vi "Periodic Tasks Gear.vi"(8 "error in":errorcluster) -> ()   [LabVIEW 2016]
uses:
  <userlib>/836-libraries/Drive/Drive_Code/Drive_Code_Support/Drive_Code_PID_Bundle.ctl
  <vilib>/Platform/TimedLoop/XDataNode/timing_clust.ctl
  <vilib>/Platform/TimedLoop/XDataNode/nitl_modes.ctl
  <vilib>/Platform/TimedLoop/XDataNode/wakeup.ctl
  <vilib>/Rock Robotics/WPI/RobotDrive/WPI_RobotDriveDevRef.ctl
  <vilib>/Rock Robotics/WPI/MotorControl/WPI_MotorControlDeviceRef.ctl
  <vilib>/Rock Robotics/WPI/MotorControl/WPI_MotorControlType.ctl
  <vilib>/Rock Robotics/SystemInterfaces/DIO/FPGA_DIOPWMChannel.ctl
  <vilib>/Rock Robotics/WPI/PWM/WPI_PWMDeadband.ctl
  <vilib>/Rock Robotics/WPI/ThirdParty/CanMotor/TalonSRX/WPI_CANTalonSRX_APIControlMode.ctl
  <vilib>/Rock Robotics/WPI/Utilities/WPI_GetSetVariantRefNum.vi
  <vilib>/addons/control/pid/pid.llb/PID (DBL).vi
  <vilib>/platform/TimedLoop/XDataNode/XDataNode.xnode
  <vilib>/Platform/TimedLoop/XDataNode/XDNodeRunTimeDep.lvlib
  <vilib>/addons/control/pid/NI_PID_pid.lvlib
panel:
  in  "PID gains 2":T1={"proportional gain (Kc)"=0.08, "integral time (Ti, min)"=0.0, "derivative time (Td, min)"=0.001} {"derivative time (Td, min)" format="%.3f"; "integral time (Ti, min)" format="%.3f"; "proportional gain (Kc)" format="%.3f"}
  in  "Offset":dbl=30.0
  in  "Max Throttle":dbl=0.4
  in  "Negate":bool=TRUE
  in  "Follow Cam":bool=TRUE
  in  "reset":bool
  in  "PID Gains 2":T2={"Yaw, Driving Straight"={"proportional gain (Kc)"=0.035, "integral time (Ti, min)"=0.0, "derivative time (Td, min)"=0.0008}, "Yaw, Holding Still"={"proportional gain (Kc)"=0.0, "integral time (Ti, min)"=0.0, "derivative time (Td, min)"=0.0}, "Distance, Driving Straight"={"proportional gain (Kc)"=0.0, "integral time (Ti, min)"=0.0, "derivative time (Td, min)"=0.0}, "Distance, Holding Still"={"proportional gain (Kc)"=0.0, "integral time (Ti, min)"=0.0, "derivative time (Td, min)"=0.0}}
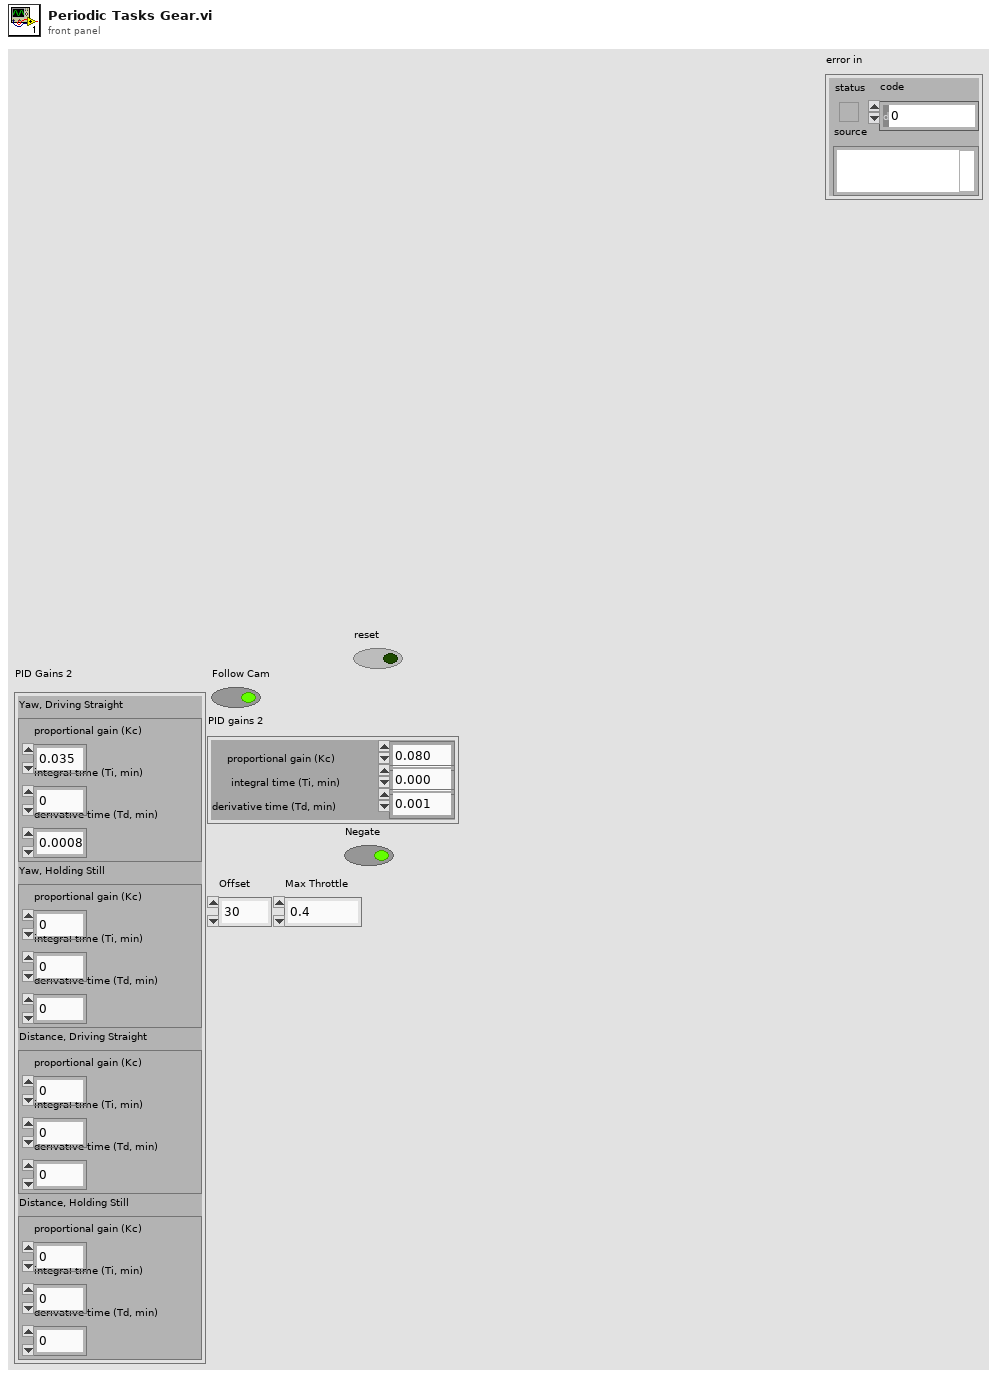
[diagram p1: front panel]
types:
  T1 = cluster{"proportional gain (Kc)":dbl, "integral time (Ti, min)":dbl, "derivative time (Td, min)":dbl}
  T2 = typedef "Drive_Code_PID_Bundle.ctl" = cluster{"Yaw, Driving Straight":cluster{"proportional gain (Kc)":dbl, "integral time (Ti, min)":dbl, "derivative time (Td, min)":dbl}, "Yaw, Holding Still":cluster{"proportional gain (Kc)":dbl, "integral time (Ti, min)":dbl, "derivative time (Td, min)":dbl}, "Distance, Driving Straight":cluster{"proportional gain (Kc)":dbl, "integral time (Ti, min)":dbl, "derivative time (Td, min)":dbl}, "Distance, Holding Still":cluster{"proportional gain (Kc)":dbl, "integral time (Ti, min)":dbl, "derivative time (Td, min)":dbl}}
  T3 = typedef "WPI_RobotDriveDevRef.ctl" = cluster{"DevStatus":errorcluster, "Motors[]":T4[], "Square Inputs":bool, "Max Output":dbl}
  T4 = typedef "WPI_MotorControlDeviceRef.ctl" = cluster{"DeviceStatus":errorcluster, "Type":T5, "PWM":cluster{"PWM Channel":T6, "DeadBand":T7}, "CAN":cluster{"Device Number":u8, "SetOutput VI Ref":variant, "GetOutput VI Ref":variant, "Enable VI Ref":variant, "Disable VI Ref":variant, "Data":variant}, "Invert":bool}
  T5 = typedef "WPI_MotorControlType.ctl" = enum16{"PWM", "CAN"}
  T6 = typedef "FPGA_DIOPWMChannel.ctl" = enum8{"PWM 0", "PWM 1", "PWM 2", "PWM 3", "PWM 4", "PWM 5", "PWM 6", "PWM 7", "PWM 8", "PWM 9", "PWM MXP 0", "PWM MXP 1", "PWM MXP 2", "PWM MXP 3", "PWM MXP 4", "PWM MXP 5", "PWM MXP 6", "PWM MXP 7", "PWM MXP 8", "PWM MXP 9", "Invalid"}
  T7 = typedef "WPI_PWMDeadband.ctl" = cluster{"Name":string, "maxPositivePwm":i32, "minPositivePwm":i32, "centerPwm":i32, "maxNegativePwm":i32, "minNegativePwm":i32, "angularRange":u16}
  T8 = typedef "Drive_Code_Bundle.ctl" = cluster{"Sensor Data":T9, "Drive Command rt fifo":refnum<k33>, "Logging Data":refnum<k33>}
  T9 = typedef "Sensor_Cluster.ctl" = cluster{"Gyro Data":cluster{"Gyro RT FIFO":refnum<k33>, "Gyro Current":dbl, "Gyro Hold":dbl}, "Encoder Data":cluster{"Encoder RT FIFO":refnum<k33>, "Encoder Current":dbl, "Encoder Hold":dbl}, "Camera Data":cluster{"Camera RT FIFO":refnum<k33>, "Camera Current":T10}}
  T10 = typedef "Camera_Cluster.ctl" = cluster{" Angle":dbl, "Valid":bool}
  T11 = typedef "WPI_EncoderDevRef.ctl" = cluster{"DevStatus":errorcluster, "EncoderIndex":T12, "CounterIndex":T13, "DistancePerCount":dbl, "Decoding Type":T14}
  T12 = typedef "FPGA_EncoderIdx.ctl" = enum8{"Enc 0", "Enc 1", "Enc 2", "Enc 3", "Enc 4", "Enc 5", "Enc 6", "Enc 7", "Invalid"}
  T13 = typedef "FPGA_CounterCtrSystemIndex.ctl" = enum8{"Ctr 0", "Ctr 1", "Ctr 2", "Ctr 3", "Ctr 4", "Ctr 5", "Ctr 6", "Ctr 7", "Invalid"}
  T14 = typedef "WPI_EncoderType.ctl" = enum16{"1x", "2x", "4x"}
  T15 = typedef "WPI_I2CDevRef.ctl" = cluster{"DevStatus":errorcluster, "Device Address":u8, "Handle":i32, "I2C Bus":T16}
  T16 = typedef "i2c_bus.ctl" = enum16{"I2C On-Board", "I2C MXP", "Invalid"}
  T17 = typedef "XDNodeRunTimeDep.lvlib/timing_clust.ctl" = cluster{"Expected End [f-1]":u64, "Actual End [f-1]":u64, "Finished Late? [f-1]":bool, "Expected End [i-1]":u64, "Actual End [i-1]":u64, "Finished Late? [i-1]":bool, "Expected Start [i]":u64, "Actual Start [i]":u64, "Expected Start [f]":u64, "Actual Start [f]":u64, "Source Name":string, "Structure Name":string, "Period":i64, "Deadline":i64, "Offset":i64, "Start":i64, "Priority":i32, "Timeout":i32, "Mode":T18, "Wakeup Reason":T19, "Error":errorcluster, "Source Type":string, "Secondary Source Type":string, "Global End Time":u64, "Global Start Time":u64, "Frame Duration":u64, "Iteration Duration":u64, "Assigned CPU":i32, "I/O Scan Engine Mode":u32}
  T18 = typedef "XDNodeRunTimeDep.lvlib/nitl_modes.ctl" = enum32{"No Change", "Process missed periods, maintain original phase", "Discard missed periods, maintain original phase", "Process missed periods, ignore original phase", "Discard missed periods, ignore original phase"}
  T19 = typedef "XDNodeRunTimeDep.lvlib/wakeup.ctl" = enum32{"Normal", "Aborted", "Asynchronous wakeup", "Timing source error", "Timed loop error", "Timeout"}
  T20 = typedef "WPI_JoystickDevRef.ctl" = cluster{"Device":T21}
  T21 = typedef "WPI_JoystickDeviceEnum.ctl" = enum16{"USB 0", "USB 1", "USB 2", "USB 3", "USB 4", "USB 5"}
  T22 = cluster{"Yaw":dbl, "Roll":dbl, "Pitch":dbl, "Yaw Wind":dbl, "Roll Wind":dbl, "Pitch Wind":dbl}
  T23 = typedef "WPI_CANTalonSRX_APIControlMode.ctl" = enum8{"Percent VBus", "Speed", "Position", "Slave", "Unchanged / Invalid", "Voltage Compensation", "Current", "Motion Profile", "Motion Magic"}
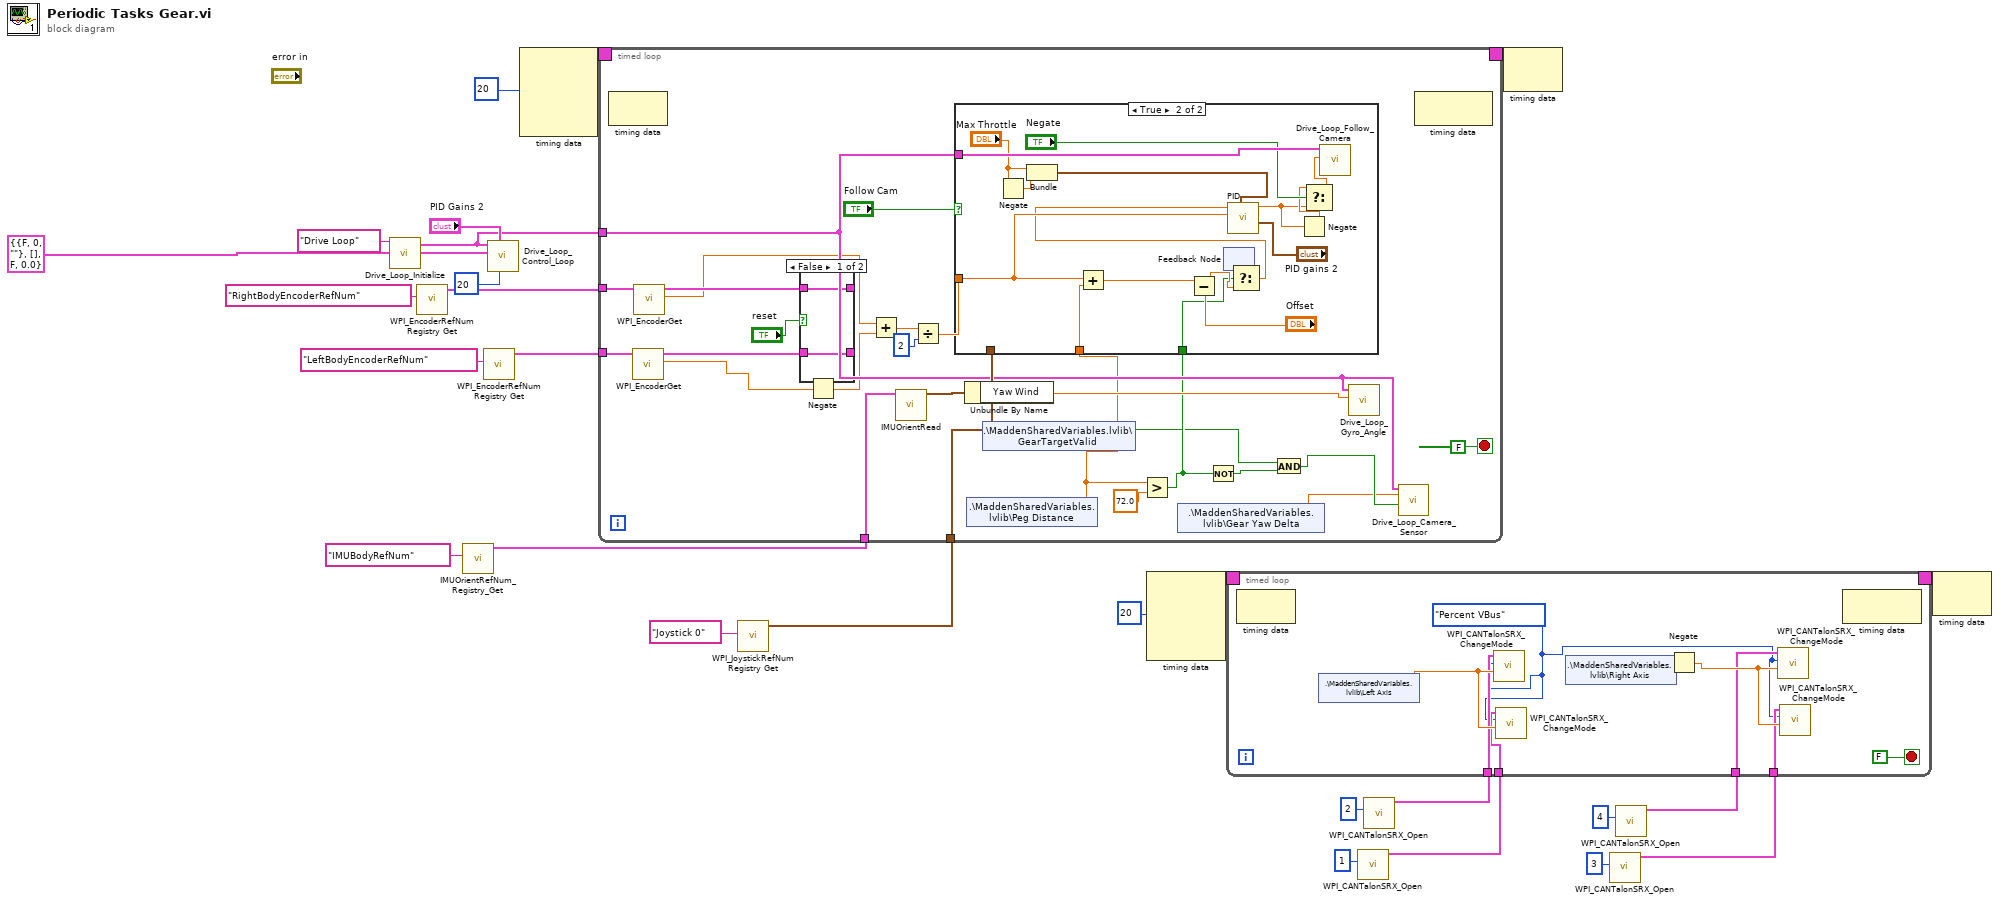
[diagram p0: block diagram]
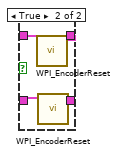
[diagram p2: hidden frame]
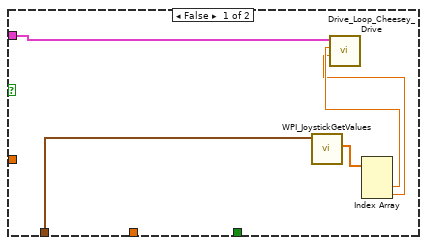
[diagram p3: hidden frame]
diagram:
  n1 = call <userlib>:"Drive_Loop_Initialize.vi"("Name of drive loop (give it a name!)"="Drive Loop") -> ("Drive Loop Cluster"=w20:T8)  [unwired: 9 in, 1 out]
  n2 = call <vilib>:"WPI_EncoderRefNum Registry Get.vi"("refnum name"="RightBodyEncoderRefNum") -> ("EncoderDevRef"=w12:T11)  [unwired: 9 in, 1 out]
  n3 = call <userlib>:"IMUOrientRefNum_Registry_Get.vi"("refnum name"="IMUBodyRefNum") -> ("I2CDevRef out"=w17:T15)  [unwired: 9 in, 1 out]
  n4 = call <vilib>:"WPI_EncoderRefNum Registry Get.vi"("refnum name"="LeftBodyEncoderRefNum") -> ("EncoderDevRef"=w11:T11)  [unwired: 9 in, 1 out]
  n5 = call <userlib>:"Drive_Loop_Control_Loop.vi"("Period \n- Amount of time between iterations of the timed control loop"=i64 20 ("Period \n- Amount of time between iterations of the timed control loop"), "PID Gains"="PID Gains 2", "RobotDriveDevRef"=T3 {"DevStatus"={"status"=FALSE, "code"=0, "source"=""}, "Motors[]"=[], "Square Inputs"=FALSE, "Max Output"=0.0}, "Control Cluster"=w20) -> ()  [unwired: 8 in]
  n6 = node-c288(i64 20 ("Period")) -> (w27:T17)  [unwired: 3 in]
  n7 = call <vilib>:"WPI_JoystickRefNum Registry Get.vi"("refnum name"="Joystick 0") -> ("JoystickDevRef"=w15:T20)  [unwired: 9 in, 1 out]
  n8 = timed-loop {
    tunnel: w20 -> [w47]
    timing: w27 -> [_]
    timing-out: [_] -> w26
    tunnel: w17 -> [w50]
    tunnel: w15 -> [w48]
    tunnel: w12 -> [w46]
    tunnel: w11 -> [w45]
    stop <- FALSE stop-if-true
    n9 = node-c288() -> ()  [unwired: 1 in, 1 out]
    n10 = call <vilib>:"WPI_EncoderGet.vi"("EncoderDevRef"=w45) -> ("Distance"=w29:dbl, "EncoderDevRef"=w43:T11)  [unwired: 5 in, 4 out]
    n11 = call <vilib>:"WPI_EncoderGet.vi"("EncoderDevRef"=w46) -> ("Distance"=w30:dbl, "EncoderDevRef"=w44:T11)  [unwired: 5 in, 4 out]
    n12 = case shown="False" "reset" {
      tunnel: w44 -> [w54 w58]
      tunnel: w43 -> [w53 w55]
      tunnel: [w54 w57] -> _
      tunnel: [w53 w56] -> _
      frame False {
      }
      frame True {
        n13 = call <vilib>:"WPI_EncoderReset.vi"("EncoderDevRef"=w58) -> ("EncoderDevRef"=w57:T11)  [unwired: 9 in, 1 out]
        n14 = call <vilib>:"WPI_EncoderReset.vi"("EncoderDevRef"=w55) -> ("EncoderDevRef"=w56:T11)  [unwired: 9 in, 1 out]
      }
    }
    n15 = Negate(x=w29) -> (-x=w31:dbl)
    n16 = Add(x=w30, y=w31) -> (x+y=w40:dbl)
    n17 = call <userlib>:"IMUOrientRead.vi"("I2CDevRef"=w50) -> ("Orient Y/R/P"=w49:T22)  [unwired: 8 in, 6 out]
    n18 = Divide(x=w40, y=2) -> (x/y=w39:dbl)
    n19 = Unbundle By Name(w49) -> ("Yaw Wind"=w38:dbl)
    n20 = shared-variable ".\\MaddenSharedVariables.lvlib\\Peg Distance"() -> (w36:dbl)  [unwired: 1 in, 1 out]
    n21 = shared-variable ".\\MaddenSharedVariables.lvlib\\GearTargetValid"() -> (w33:bool)  [unwired: 1 in, 1 out]
    n22 = Greater?(x=w36, y=72.0) -> (0:w35:bool)
    n23 = case shown="True" "Follow Cam" {
      tunnel: w47 -> [w63 w80]
      tunnel: w48 -> [w62 _]
      tunnel: w39 -> [_ w70]
      tunnel: w36 -> [_ w65]
      tunnel: w35 -> [_ w64]
      frame False {
        n24 = call <vilib>:"WPI_JoystickGetValues.vi"("JoystickDevRef"=w62) -> ("Axes"=w61:dbl[])  [unwired: 6 in, 4 out]
        n25 = Index Array(array=w61) -> (element #2=w60:dbl, element #3=w59:dbl)  [unwired: 3 in, 1 out]
        n26 = call <userlib>:"Drive_Loop_Cheesey_Drive.vi"("Wheel"=w59, "Throttle"=w60, "Drive Loop Cluster"=w63) -> ()  [unwired: 9 in]
      }
      frame True {
        n27 = Negate(x="Max Throttle") -> (-x=w76:dbl)
        n28 = Bundle("Max Throttle"="Max Throttle", w76) -> (w75:cluster{"Max Throttle":dbl, dbl})  [unwired: 1 in]
        n29 = Add(x=w70, y=w65) -> (x+y=w78:dbl)
        n30 = Subtract(x=w78, y="Offset") -> (x-y=w68:dbl)
        n31 = feedback #1() -> (w67:dbl)  [unwired: 1 in]
        n32 = Select(t=w67, s=w64, f=w68) -> (s? t:f=w66:dbl)
        n33 = feedback-in #1(w66) -> ()
        n34 = call-poly <vilib>:"PID.vi"("output range"=w75, "PID gains"="PID gains 2", "process variable"=w70, "setpoint"=w66) -> ("output"=w72:dbl)  [unwired: 6 in, 1 out]
        n35 = Negate(x=w72) -> (-x=w73:dbl)
        n36 = Select(t=w73, s="Negate", f=w72) -> (s? t:f=w71:dbl)
        n37 = call <userlib>:"Drive_Loop_Follow_Camera.vi"("Power Level #6"=w71, "Drive Loop Cluster"=w80) -> ()  [unwired: 10 in]
      }
    }
    n38 = shared-variable ".\\MaddenSharedVariables.lvlib\\Gear Yaw Delta"() -> (w28:dbl)  [unwired: 1 in, 1 out]
    n39 = Not(x=w35) -> (.not. x?=w34:bool)
    n40 = And(x=w33, y=w34) -> (x .and. y?=w32:bool)
    n41 = call <userlib>:"Drive_Loop_Gyro_Angle.vi"("Yaw Wind"=w38, "Drive Loop Cluster"=w47) -> ()  [unwired: 10 in]
    n42 = call <userlib>:"Drive_Loop_Camera_Sensor.vi"("Stable?"=w32, "Camera Angle"=w28, "Drive Loop Cluster"=w47) -> ()  [unwired: 9 in]
    n43 = node-c288() -> ()  [unwired: 1 in, 1 out]
  }
  n44 = node-c288(i64 20 ("Period")) -> (w25:T17)  [unwired: 3 in]
  n45 = call <vilib>:"WPI_CANTalonSRX_Open.vi"("Device Number"=u8 1) -> ("CAN Talon SRX Ref"=w7:T4)  [unwired: 9 in, 1 out]
  n46 = call <vilib>:"WPI_CANTalonSRX_Open.vi"("Device Number"=u8 2) -> ("CAN Talon SRX Ref"=w8:T4)  [unwired: 9 in, 1 out]
  n47 = node-c288(w26) -> ()  [unwired: 1 out]
  n48 = call <vilib>:"WPI_CANTalonSRX_Open.vi"("Device Number"=u8 3) -> ("CAN Talon SRX Ref"=w9:T4)  [unwired: 9 in, 1 out]
  n49 = call <vilib>:"WPI_CANTalonSRX_Open.vi"("Device Number"=u8 4) -> ("CAN Talon SRX Ref"=w10:T4)  [unwired: 9 in, 1 out]
  n50 = timed-loop {
    timing: w25 -> [_]
    timing-out: [_] -> w24
    tunnel: w10 -> [w88]
    tunnel: w9 -> [w87]
    tunnel: w8 -> [w86]
    tunnel: w7 -> [w85]
    stop <- FALSE stop-if-true
    w84 = WPI_CANTalonSRX_APIControlMode."Percent VBus" ("Control Mode")
    n51 = node-c288() -> ()  [unwired: 1 in, 1 out]
    n52 = shared-variable ".\\MaddenSharedVariables.lvlib\\Left Axis"() -> (w90:dbl)  [unwired: 1 in, 1 out]
    n53 = call <vilib>:"WPI_CANTalonSRX_ChangeMode.vi"("Output"=w90, "Control Mode"=w84, "CAN Talon SRX Ref"=w86) -> ()  [unwired: 7 in, 2 out]
    n54 = call <vilib>:"WPI_CANTalonSRX_ChangeMode.vi"("Output"=w90, "Control Mode"=w84, "CAN Talon SRX Ref"=w85) -> ()  [unwired: 7 in, 2 out]
    n55 = shared-variable ".\\MaddenSharedVariables.lvlib\\Right Axis"() -> (w91:dbl)  [unwired: 1 in, 1 out]
    n56 = Negate(x=w91) -> (-x=w89:dbl)
    n57 = call <vilib>:"WPI_CANTalonSRX_ChangeMode.vi"("Output"=w89, "Control Mode"=w84, "CAN Talon SRX Ref"=w88) -> ()  [unwired: 7 in, 2 out]
    n58 = call <vilib>:"WPI_CANTalonSRX_ChangeMode.vi"("Output"=w89, "Control Mode"=w84, "CAN Talon SRX Ref"=w87) -> ()  [unwired: 7 in, 2 out]
    n59 = node-c288() -> ()  [unwired: 1 in, 1 out]
  }
  n60 = node-c288(w24) -> ()  [unwired: 1 out]
